vi "read IO variable U32.vi"(8 "error in (no error)":errorcluster, 9 "data type":u32, 10 "IO Variable":T1=4 items=["Control Word", "Target Position", "Target Torque", "Target Velocity", "Position Actual Value", "Status Word", "Torque Actual Value", "Velocity Actual Value"], 11 "IO variable Array In":refnum<k21>[](array[refnum])) -> (0 "error out":errorcluster, 2 "data out":u32, 3 "IO variable Array Out":refnum<k21>[](array[refnum]))   [LabVIEW 2016, in "Scan Engine Custom Device.lvlib" / "DS402.lvlib"]
uses:
  DS402.lvlib
  controls/IOvariables.ctl
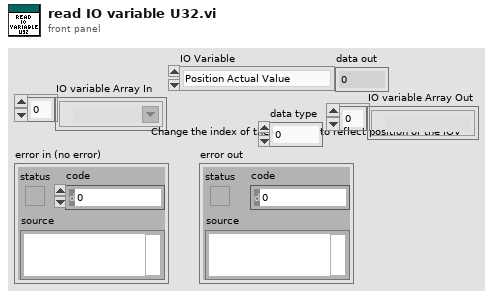
[diagram p1: front panel]
types:
  T1 = typedef "Scan Engine Custom Device.lvlib/DS402.lvlib/IOvariables.ctl" = u16
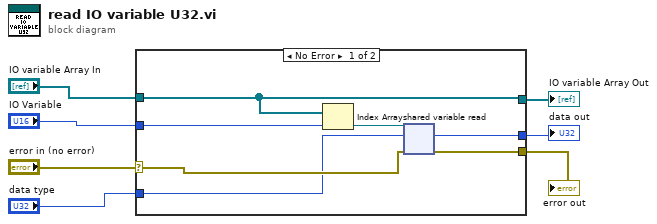
[diagram p0: block diagram]
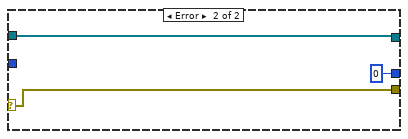
[diagram p2: hidden frame]
diagram:
  n1 = case shown="No Error" "error in (no error)" {
    selector: "error in (no error)" -> [w13 w17]
    tunnel: [w12 w17] -> w6
    tunnel: "IO Variable" -> [w11 _]
    tunnel: "data type" -> [w10 _]
    tunnel: "IO variable Array In" -> [w9 w16]
    tunnel: [w9 w16] -> w2
    tunnel: [w8 u32 0 ("data type")] -> w1
    frame No Error {
      n2 = Index Array(array=w9, index=w11) -> (element=w14:refnum<k21>)
      n3 = shared-variable-read(w14, w13, w10) -> (w12:errorcluster, w8:u32)  [unwired: 2 out]
    }
    frame Error {
    }
  }
  "error out" <- w6
  "IO variable Array Out" <- w2
  "data out" <- w1
